vi "EZ Totalizer.vi"(8 "error in (no error)":errorcluster, 9 "Read/R-Reset (F:Read)":bool, 10 "Scan List (empty)":string, 11 "VISA Resource Name":refnum<visa-resource-name>) -> (0 "error out":errorcluster, 2 "Output Array":u32[](array[numeric]), 3 "VISA Resource Name Out":refnum<visa-resource-name>)   [LabVIEW 2016, in "Agilent 34970.lvlib"]
doc: "This VI lets you take simple totalizer readings."
uses:
  Agilent 34970.lvlib
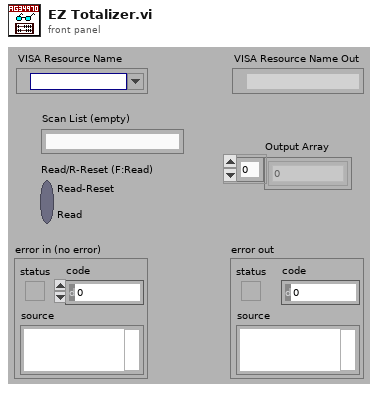
[diagram p1: front panel]
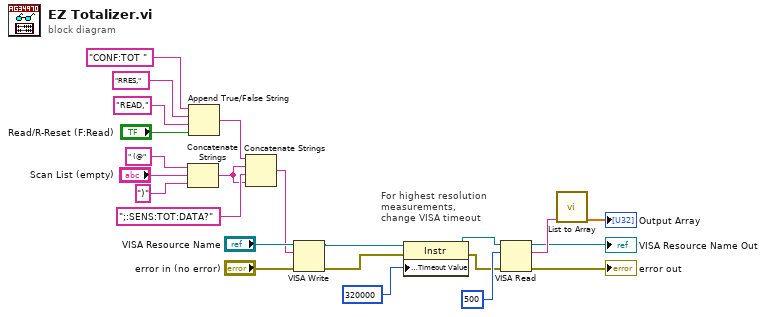
[diagram p0: block diagram]
diagram:
  # "For highest resolution\nmeasurements, \nchange VISA timeout"
  n1 = Concatenate Strings(" (@", "Scan List (empty)", ")") -> (w6:string)
  n2 = Append True/False String(1:"Read/R-Reset (F:Read)", 2:"READ,", 3:"RRES,", 4:"CONF:TOT ") -> (0:w9:string)
  n3 = Concatenate Strings(w9, w6, ";:SENS:TOT:DATA?", w6) -> (w8:string)
  n4 = VISA Write(VISA resource name="VISA Resource Name", write buffer=w8, error in (no error)="error in (no error)") -> (VISA resource name out=w4:refnum<visa-resource-name>, error out=w3:errorcluster)  [unwired: 1 out]
  n5 = property class="Instr"(reference=w4, error in=w3, "General Settings:Timeout Value"=u32 320000 ("Tmo Value")) -> (reference out=w2:refnum<visa-resource-name>, error out=w1:errorcluster)
  n6 = VISA Read(VISA resource name=w2, byte count=u32 500 ("byte count (0)"), error in (no error)=w1) -> (VISA resource name out=→"VISA Resource Name Out":refnum<visa-resource-name>, read buffer=w16:string, error out=→"error out":errorcluster)  [unwired: 1 out]
  n7 = call "List to Array.vi"("List (empty)"=w16) -> ("Output Number Array"=→"Output Array":dbl[])  [unwired: 9 in, 1 out]
